vi "Set carrier freq - Tx.vi"(8 "error in (no error)":errorcluster, 10 "Carrier freq [MHz]":dbl, 11 "FpgaRefx410 in":refnum<class "FpgaRefx410.lvclass">) -> (0 "error out":errorcluster, 3 "FpgaRefx410 out":refnum<class "FpgaRefx410.lvclass">)   [LabVIEW 2025, in "FpgaRefx410.lvclass"]
uses:
  FpgaRefx410.lvclass
  FpgaRefx410.lvclass/FpgaRefx410.ctl
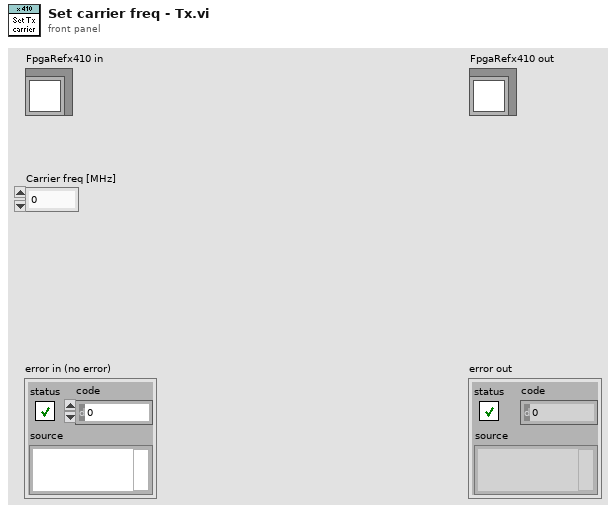
[diagram p1: front panel]
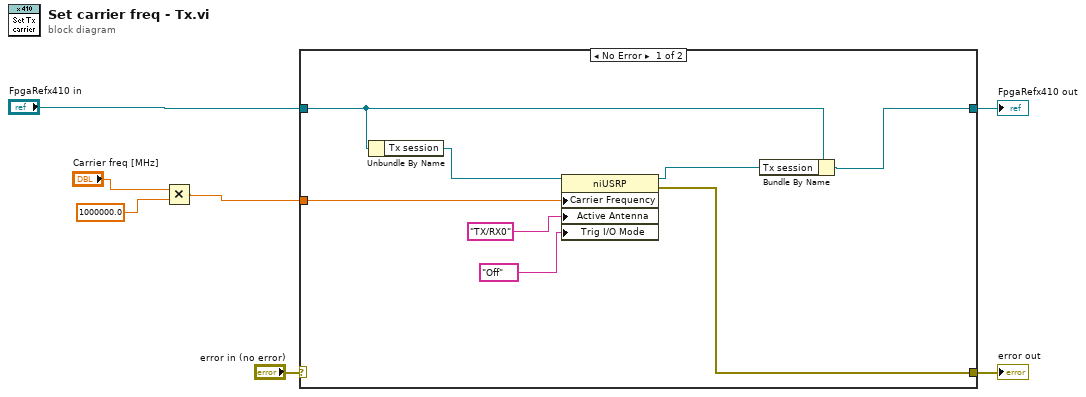
[diagram p0: block diagram]
diagram:
  n1 = Multiply(x="Carrier freq [MHz]", y=1000000.0) -> (x*y=w1:dbl)
  n2 = case shown="No Error" "error in (no error)" {
    selector: "error in (no error)" -> [_ w17]
    tunnel: [w9 w17] -> w6
    tunnel: [w8 w16] -> w4
    tunnel: "FpgaRefx410 in" -> [w11 w16]
    tunnel: w1 -> [w12 _]
    frame No Error {
      n3 = Unbundle By Name(w11) -> ("Tx session"=w13:refnum<k15>)
      n4 = property class="niUSRP"(reference=w13, "Carrier Frequency"=w12, "Active Antenna"="TX/RX0" ("Configuration:Active Antenna"), "Trig I/O Mode"="Off" ("Configuration:Trig I/O Mode")) -> (reference out=w10:refnum<k15>, error out=w9:errorcluster)  [unwired: 1 in]
      n5 = Bundle By Name(cluster=w11, "Tx session"=w10) -> (w8:refnum<class "FpgaRefx410.lvclass">)
    }
    frame Error {
    }
  }
  "error out" <- w6
  "FpgaRefx410 out" <- w4
